vi "Pulse.vi"(10 "Pulse":i32=100) -> (2 "Pulse":string)   [LabVIEW 2017]
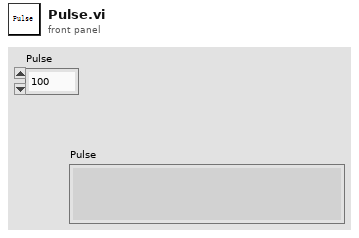
[diagram p1: front panel]
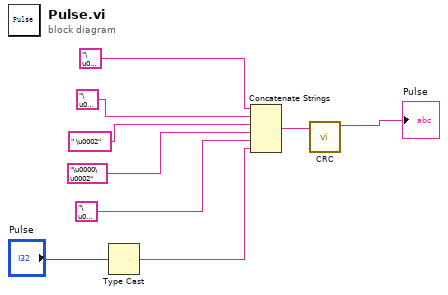
[diagram p0: block diagram]
diagram:
  n1 = Type Cast(x="Pulse") -> (*(type *) &x=w1:string)  [unwired: 1 in]
  n2 = Concatenate Strings("\u0001", "\u0010", " \u0002", "\u0000\u0002", "\u0004", w1) -> (w5:string)
  n3 = call "CRC.vi"("字符串"=w5) -> ("连接的字符串"=→"Pulse":string)  [unwired: 9 in, 1 out]
